vi "Read Settings.vi"(8 "error in (no error)":errorcluster, 11 "EGG7280 in":refnum<class "EGG7280.lvclass">) -> (0 "error out":errorcluster, 2 "Settings":string, 3 "EGG7280 out":refnum<class "EGG7280.lvclass">)   [LabVIEW 2015, in "EGG7280.lvclass"]
uses:
  EGG7280.lvclass
  Instrument/Instrument.lvclass
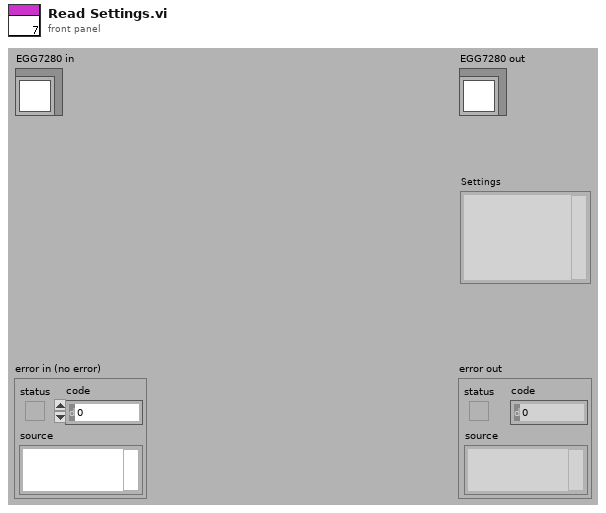
[diagram p1: front panel]
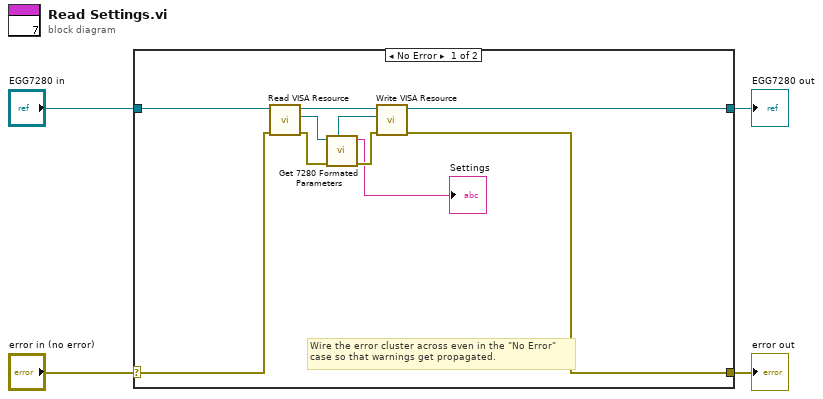
[diagram p0: block diagram]
diagram:
  n1 = case shown="No Error" "error in (no error)" {
    selector: "error in (no error)" -> [w10 w16]
    tunnel: [w7 w16] -> w3
    tunnel: [w12 w15] -> w1
    tunnel: "EGG7280 in" -> [w13 w15]
    frame No Error {
      # "Wire the error cluster across even in the \"No Error\"\ncase so that warnings get propagated."
      n2 = call "Read VISA Resource.vi"("error in (no error)"=w10, "Instrument.lvclass in"=w13) -> ("error out"=w9:errorcluster, "VISA Resource"=w11:refnum<visa-resource-name>, "Instrument.lvclass out"=w14:refnum<class "EGG7280.lvclass">)  [unwired: 7 out]
      n3 = call "Get 7280 Formated Parameters.VI"("error in (no error)"=w9, "VISA Resource Name"=w11) -> ("error out"=w8:errorcluster, "Parameters"=→"Settings":string, "VISA Resource Name Out"=w6:refnum<visa-resource-name>)  [unwired: 1 in, 6 out]
      n4 = call "Write VISA Resource.vi"("error in (no error)"=w8, "VISA Resource"=w6, "Instrument.lvclass in"=w14) -> ("error out"=w7:errorcluster, "Instrument.lvclass out"=w12:refnum<class "EGG7280.lvclass">)  [unwired: 7 out]
    }
    frame Error {
    }
  }
  "error out" <- w3
  "EGG7280 out" <- w1
